vi "Vision-Goal.vi"() -> (12 "Goal Detected":bool, 14 "Goal Angle (radians 0=right)":dbl, 15 "Goal Distance (from front of shooter)":dbl)   [LabVIEW 2015]
uses:
  labview-zmq/socket_type.ctl
  labview-zmq/socket_options.ctl
  labview-zmq/zmq_socket.lvclass
  labview-zmq/zmq_context.lvclass
  labview-zmq/zeromq.lvlib
  <vilib>/Rock Robotics/Network Tables/NT Read Number.vi
panel:
  in  "Boolean":bool
  out "data 2":string
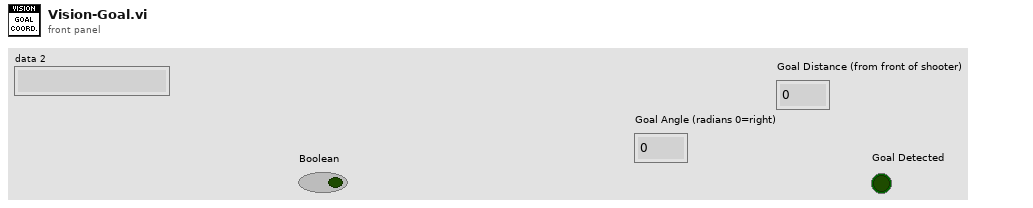
[diagram p1: front panel]
types:
  T1 = typedef "zeromq.lvlib/socket_options.ctl" = enum8{"NONE", "ZMQ_HWM", "<2>", "ZMQ_SWAP", "ZMQ_AFFINITY", "ZMQ_IDENTITY", "ZMQ_SUBSCRIBE", "ZMQ_UNSUBSCRIBE", "ZMQ_RATE", "ZMQ_RECOVERY_IVL", "ZMQ_MCAST_LOOP", "ZMQ_SNDBUF", "ZMQ_RCVBUF", "ZMQ_RCVMORE", "ZMQ_FD", "ZMQ_EVENTS", "ZMQ_TYPE", "ZMQ_LINGER", "ZMQ_RECONNECT_IVL", "ZMQ_BACKLOG", "ZMQ_RECOVERY_IVL_MSEC", "ZMQ_RECONNECT_IVL_MAX", "ZMQ_MAXMSGSIZE", "ZMQ_SNDHWM", "ZMQ_RCVHWM", "ZMQ_MULTICAST_HOPS", "<26>", "ZMQ_RCVTIMEO", "ZMQ_SNDTIMEO", "<29>", "<30>", "ZMQ_IPV4ONLY", "ZMQ_LAST_ENDPOINT", "ZMQ_ROUTER_MANDATORY", "ZMQ_TCP_KEEPALIVE", "ZMQ_TCP_KEEPALIVE_CNT", "ZMQ_TCP_KEEPALIVE_IDLE", "ZMQ_TCP_KEEPALIVE_INTVL", "ZMQ_TCP_ACCEPT_FILTER", "ZMQ_DELAY_ATTACH_ON_CONNECT", "ZMQ_XPUB_VERBOSE"}
  T2 = typedef "zeromq.lvlib/socket_type.ctl" = enum8{"ZMQ_PAIR", "ZMQ_PUB", "ZMQ_SUB", "ZMQ_REQ", "ZMQ_REP", "ZMQ_DEALER", "ZMQ_ROUTER", "ZMQ_PULL", "ZMQ_PUSH", "ZMQ_XPUB", "ZMQ_XSUB"}
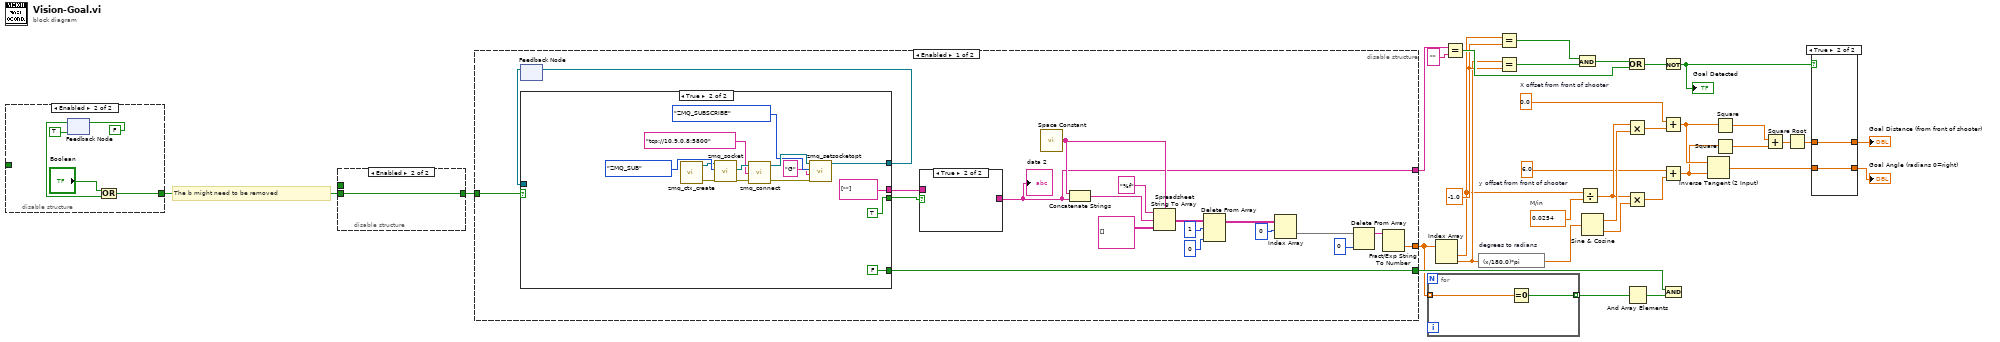
[diagram p0: block diagram]
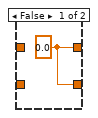
[diagram p2: hidden frame]
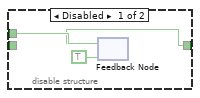
[diagram p3: hidden frame]
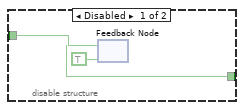
[diagram p4: hidden frame]
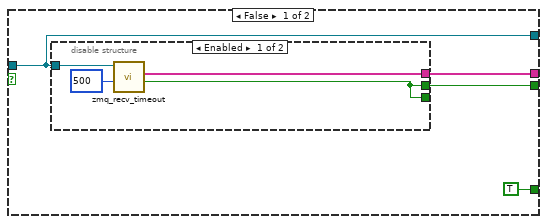
[diagram p5: hidden frame]
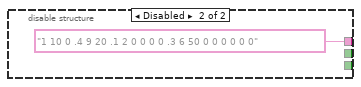
[diagram p6: hidden frame]
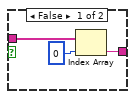
[diagram p7: hidden frame]
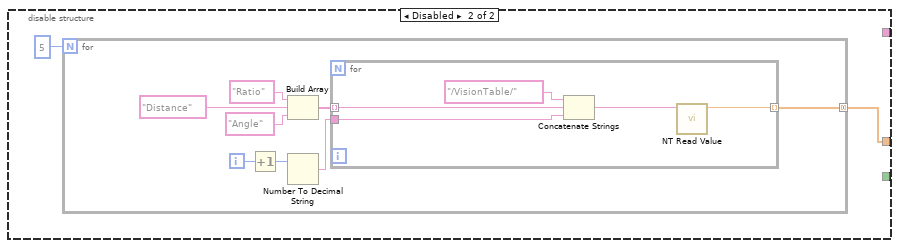
[diagram p8: hidden frame]
diagram:
  w18 = 6.0  # y offset from front of shooter
  w19 = 0.0  # X offset from front of shooter
  w31 = 0.0254  # M/in
  w6 = -1.0 ("y")
  # "The b might need to be removed"
  n1 = disable-structure shown="Enabled" {
    disable-tunnel: _ -> [w38 _]
    disable-tunnel: [w36 w41] -> w13
    frame Disabled {
      n2 = feedback #1(TRUE) -> (w36:bool)
      n3 = feedback-in #1(w38) -> ()
    }
    frame Enabled {
      n4 = feedback-in #2(FALSE) -> ()
      n5 = feedback #2(TRUE) -> (w40:bool)
      n6 = Or(x="Boolean", y=w40) -> (x .or. y?=w41:bool)
    }
  }
  n7 = disable-structure shown="Enabled" {
    disable-tunnel: _ -> [w46 _]
    disable-tunnel: [w44 w47] -> w32
    disable-tunnel: w13 -> [_ w47]
    frame Disabled {
      n8 = feedback #3(TRUE) -> (w44:bool)
      n9 = feedback-in #3(w46) -> ()
    }
    frame Enabled {
    }
  }
  n10 = disable-structure shown="Enabled" {
    disable-tunnel: [w62 w95] -> w12
    disable-tunnel: w32 -> [w54 _]
    disable-tunnel: [w55 _] -> w33
    disable-tunnel: [w53 _] -> w17
    frame Enabled {
      n11 = feedback #4() -> (w56:refnum<class "zmq_socket.lvclass">)  [unwired: 1 in]
      n12 = case shown="True" w54 {
        tunnel: [w71 string[] [""] ("parts")] -> w59
        tunnel: [w70 TRUE ("timeout?")] -> w58
        tunnel: w56 -> [w69 _]
        tunnel: [w69 w78] -> w57
        tunnel: [TRUE FALSE] -> w55
        frame False {
          n13 = disable-structure shown="Enabled" {
            disable-tunnel: [w75 "1 10 0 .4 9 20 .1 2 0 0 0 0 .3 6 50 0 0 0 0 0 0"] -> w71
            disable-tunnel: [w73 _] -> w70
            disable-tunnel: [w73 _] -> _
            disable-tunnel: w69 -> [w72 _]
            frame Enabled {
              n14 = call "zmq_recv_timeout.vi"("timeout (ms)"=u32 500, "socket in"=w72) -> ("timeout?"=w73:bool, "parts"=w75:string[])  [unwired: 2 in, 2 out]
            }
            frame Disabled {
            }
          }
        }
        frame True {
          n15 = call "zmq_ctx_create.vi"() -> ("error out"=w86:errorcluster, "context out"=w89:refnum<class "zmq_context.lvclass">)  [unwired: 4 in]
          n16 = call "zmq_socket.vi"("error in"=w86, "socket type"=socket_type."ZMQ_SUB", "context in"=w89) -> ("error out"=w83:errorcluster, "socket out"=w88:refnum<class "zmq_socket.lvclass">)  [unwired: 2 in, 1 out]
          n17 = call "zmq_connect.vi"("error in"=w83, "endpoint"="tcp://10.9.0.8:5800" ("Endpoint"), "socket in"=w88) -> ("error out"=w84:errorcluster, "socket out"=w85:refnum<class "zmq_socket.lvclass">)  [unwired: 1 in]
          n18 = call "zmq_setsocketopt.vi"("error in"=w84, "value"="G", "option"=socket_options."ZMQ_SUBSCRIBE", "socket in"=w85) -> ("socket out"=w78:refnum<class "zmq_socket.lvclass">)  [unwired: 2 in, 1 out]
        }
      }
      n19 = feedback-in #4(w57) -> ()
      n20 = case shown="True" w58 {
        tunnel: w59 -> [w93 _]
        tunnel: [w91 _] -> w53
        frame False {
          n21 = Index Array(array=w93, index=0) -> (element=w91:string)
        }
        frame True {
        }
      }
      "data 2" <- w53
      n22 = call <vilib>:"Space Constant.vi"() -> ("String"=w60:string)
      n23 = Concatenate Strings(w60, w53) -> (w61:string)
      n24 = Spreadsheet String To Array(delimiter (Tab)=w60, format string="%f", spreadsheet string=w61, array type (2D Dbl)=string[][] [] ("Array")) -> (array=w63:string[][])
      n25 = Delete From Array(array=w63, length=1, index (col)=0 ("disabled index (col)")) -> (array with subset deleted=w52:string[][])  [unwired: 1 in, 1 out]
      n26 = Index Array(array=w52, index (row)=0) -> (element=w49:string[])  [unwired: 1 in]
      n27 = Delete From Array(array=w49, index=0) -> (array with subset deleted=w48:string[])  [unwired: 1 in, 1 out]
      n28 = Fract/Exp String To Number(string=w48) -> (number=w62:dbl[])  [unwired: 4 out]
    }
    frame Disabled {
      n29 = for {
        N: 5 -> [_]
        tunnel: [w103] -> w95 mode=concatenating
        i -> [w98]
        n30 = Increment(x=w98) -> (x+1=w97:i32)
        n31 = Build Array("Ratio" ("element"), "Distance" ("element"), "Angle") -> (w99:string[])
        n32 = Number To Decimal String(number=w97) -> (decimal integer string=w96:string)  [unwired: 1 in]
        n33 = for {
          tunnel: [w107] -> w103 mode=indexing
          tunnel: w99 -> [w106] mode=indexing
          tunnel: w96 -> [w104]
          n34 = Concatenate Strings("/VisionTable/" ("string"), w106, w104) -> (w108:string)
          n35 = call-poly <vilib>:"NT Read Value.vi"("Name"=w108) -> ("Numeric"=w107:dbl)  [unwired: 9 in, 1 out]
        }
      }
    }
  }
  n36 = for {
    tunnel: w12 -> [w110] mode=indexing
    tunnel: [w109] -> w35 mode=indexing
    n37 = Equal To 0?(x=w110) -> (x = 0?=w109:bool)
  }
  n38 = Index Array(array=w12) -> (element #1=w1:dbl, element #2=w2:dbl)  [unwired: 2 in]
  n39 = Equal?(x=w17, y="") -> (x = y?=w15:bool)
  n40 = expression code="(x/180.0)*pi" "degrees to radians"(w2) -> (w30:dbl)
  n41 = Equal?(x=w1, y=w6) -> (x = y?=w4:bool)
  n42 = Equal?(x=w2, y=w6) -> (x = y?=w5:bool)
  n43 = And(x=w4, y=w5) -> (x .and. y?=w3:bool)
  n44 = Divide(x=w1, y=w31) -> (x/y=w26:dbl)
  n45 = Sine & Cosine(0:w30) -> (1:w29:dbl, 2:w27:dbl)
  n46 = Or(x=w3, y=w15) -> (x .or. y?=w14:bool)
  n47 = Multiply(x=w26, y=w29) -> (x*y=w28:dbl)
  n48 = Multiply(x=w26, y=w27) -> (x*y=w25:dbl)
  n49 = And Array Elements(Boolean array=w35) -> (logical AND=w34:bool)
  n50 = Not(x=w14) -> (.not. x?=w7:bool)
  "Goal Detected" <- w7
  n51 = Add(x=w19, y=w28) -> (x+y=w21:dbl)
  n52 = Add(x=w18, y=w25) -> (x+y=w20:dbl)
  n53 = And(x=w33, y=w34) -> ()  [unwired: 1 out]
  n54 = Inverse Tangent (2 Input)(1:w20, 2:w21) -> (0:w10:dbl)
  n55 = Square(x=w21) -> (x^2=w24:dbl)
  n56 = Square(x=w20) -> (x^2=w23:dbl)
  n57 = Add(x=w24, y=w23) -> (x+y=w22:dbl)
  n58 = Square Root(x=w22) -> (sqrt(x)=w8:dbl)
  n59 = case shown="True" w7 {
    tunnel: [w111 w113] -> w11
    tunnel: w10 -> [_ w113]
    tunnel: [w111 w112] -> w9
    tunnel: w8 -> [_ w112]
    frame False {
      w111 = 0.0
    }
    frame True {
    }
  }
  "Goal Distance (from front of shooter)" <- w9
  "Goal Angle (radians 0=right)" <- w11
